vi "Init_Message_Queues.vi"(8 "error in (no error)":errorcluster) -> (0 "error out":errorcluster, 3 "Queue_Out":T1)   [LabVIEW 2014]
uses:
  02_Controls/Message_Queues.ctl
  02_Controls/Message_Data_Ctl.ctl
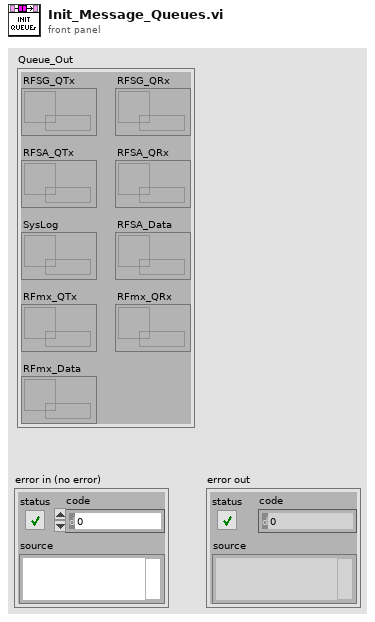
[diagram p1: front panel]
types:
  T1 = typedef "Message_Queues.ctl" = cluster{"RFSG_QTx":refnum<queue>, "RFSG_QRx":refnum<queue>, "RFSA_QTx":refnum<queue>, "RFSA_QRx":refnum<queue>, "SysLog":refnum<queue>, "RFSA_Data":refnum<queue>, "RFmx_QTx":refnum<queue>, "RFmx_QRx":refnum<queue>, "RFmx_Data":refnum<queue>}
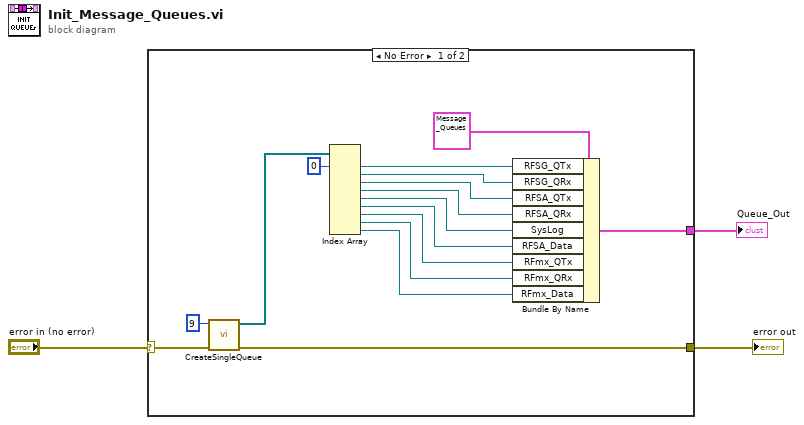
[diagram p0: block diagram]
diagram:
  n1 = case shown="No Error" "error in (no error)" {
    selector: "error in (no error)" -> [w18 w20]
    tunnel: [w17 w20] -> w2
    tunnel: [w16 _] -> w1
    frame No Error {
      n2 = call "CreateSingleQueue.vi"("Error In"=w18, "Number of Queues"=9) -> ("Error Out"=w17:errorcluster, "Q_MEMs"=w14:refnum<queue>[])  [unwired: 8 in]
      n3 = Index Array(array=w14, index #1=0 ("index")) -> (element #1=w12:refnum<queue>, element #2=w11:refnum<queue>, element #3=w10:refnum<queue>, element #4=w9:refnum<queue>, element #5=w8:refnum<queue>, element #6=w7:refnum<queue>, element #7=w6:refnum<queue>, element #8=w5:refnum<queue>, element #9=w4:refnum<queue>)  [unwired: 8 in]
      n4 = Bundle By Name(cluster=T1 {"RFSG_QTx"=refnum, "RFSG_QRx"=refnum, "RFSA_QTx"=refnum, "RFSA_QRx"=refnum, "SysLog"=refnum, "RFSA_Data"=refnum, "RFmx_QTx"=refnum, "RFmx_QRx"=refnum, "RFmx_Data"=refnum} ("Message_Queues"), "RFSG_QTx"=w12, "RFSG_QRx"=w11, "RFSA_QTx"=w10, "RFSA_QRx"=w9, "SysLog"=w8, "RFSA_Data"=w7, "RFmx_QTx"=w6, "RFmx_QRx"=w5, "RFmx_Data"=w4) -> (w16:T1)
    }
    frame Error {
    }
  }
  "error out" <- w2
  "Queue_Out" <- w1
